vi "random_subVI.vi"(1 "lower bound":dbl, 2 "upper bound":dbl) -> (0 "output":dbl)   [LabVIEW 2014]
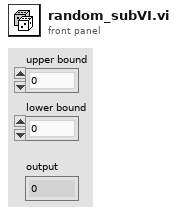
[diagram p1: front panel]
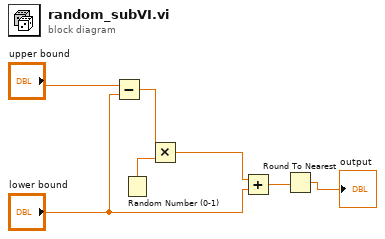
[diagram p0: block diagram]
diagram:
  n1 = Subtract(x="upper bound", y="lower bound") -> (x-y=w6:dbl)
  n2 = Random Number (0-1)() -> (number: 0 to 1=w7:dbl)
  n3 = Multiply(x=w6, y=w7) -> (x*y=w4:dbl)
  n4 = Add(x=w4, y="lower bound") -> (x+y=w2:dbl)
  n5 = Round To Nearest(number=w2) -> (nearest integer value=→"output":dbl)
